vi "Query Average.vi"(8 "Error In (no error)":errorcluster, 10 "Channel (1)":i32=1, 11 "VISA Resource Name":refnum<visa-resource-name>) -> (0 "Error Out":errorcluster, 1 "Avg count":i32, 3 "VISA Resource Name Out":refnum<visa-resource-name>)   [LabVIEW 2019]
doc: "This VI reads number of averages currntly set."
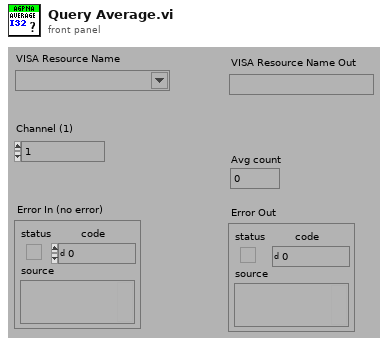
[diagram p1: front panel]
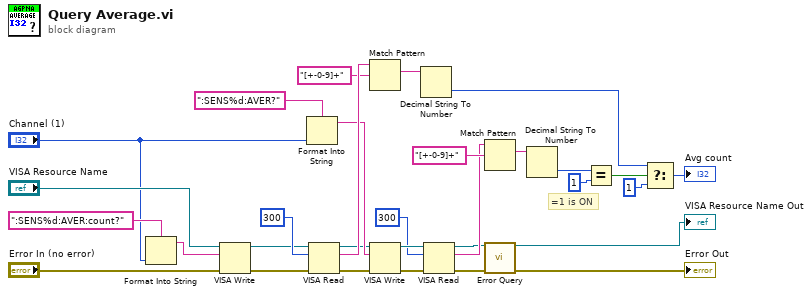
[diagram p0: block diagram]
diagram:
  # "=1 is ON"
  n1 = Format Into String(format string=":SENS%d:AVER:count?", "Channel (1)") -> (resulting string=w28:string)  [unwired: 2 in, 1 out]
  n2 = VISA Write(VISA resource name="VISA Resource Name", write buffer=w28, error in (no error)="Error In (no error)") -> (VISA resource name out=w24:refnum<visa-resource-name>, error out=w23:errorcluster)  [unwired: 1 out]
  n3 = Format Into String(format string=":SENS%d:AVER?", "Channel (1)") -> (resulting string=w13:string)  [unwired: 2 in, 1 out]
  n4 = VISA Read(VISA resource name=w24, byte count=u32 300, error in (no error)=w23) -> (VISA resource name out=w4:refnum<visa-resource-name>, read buffer=w22:string, error out=w3:errorcluster)  [unwired: 1 out]
  n5 = Match Pattern(string=w22, regular expression="[+-0-9]+") -> (match substring=w20:string)  [unwired: 1 in, 3 out]
  n6 = VISA Write(VISA resource name=w4, write buffer=w13, error in (no error)=w3) -> (VISA resource name out=w15:refnum<visa-resource-name>, error out=w16:errorcluster)  [unwired: 1 out]
  n7 = Decimal String To Number(string=w20) -> (number=w8:i32)  [unwired: 2 in, 1 out]
  n8 = VISA Read(VISA resource name=w15, byte count=u32 300, error in (no error)=w16) -> (VISA resource name out=w1:refnum<visa-resource-name>, read buffer=w17:string, error out=w2:errorcluster)  [unwired: 1 out]
  n9 = Match Pattern(string=w17, regular expression="[+-0-9]+") -> (match substring=w19:string)  [unwired: 1 in, 3 out]
  n10 = call <instrlib>:"Error Query.vi"("VISA Resource Name"=w1, "error in (no error)"=w2) -> ("VISA Resource Name Out"=→"VISA Resource Name Out":refnum<visa-resource-name>, "error out"=→"Error Out":errorcluster)  [unwired: 10 in, 2 out]
  n11 = Decimal String To Number(string=w19) -> (number=w11:i32)  [unwired: 2 in, 1 out]
  n12 = Equal?(x=w11, y=1) -> (x = y?=w9:bool)
  n13 = Select(t=w8, s=w9, f=1) -> (s? t:f=→"Avg count":i32)
